vi "PRBS64 Parallel Tx Base.vi"(6 "ready for output (T)":bool=TRUE, 7 "reset":bool, 11 "seed":u64) -> (1 "output valid":bool, 3 "prbs tx":u64)   [LabVIEW 2022 SP3, in "Aurora64b66b Utilities FPGA.lvlib"]
uses:
  Aurora64b66b Utilities FPGA.lvlib
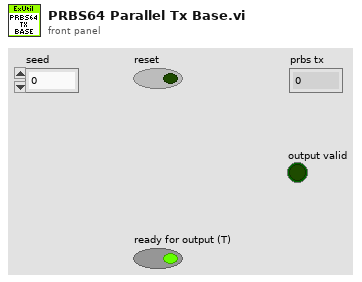
[diagram p1: front panel]
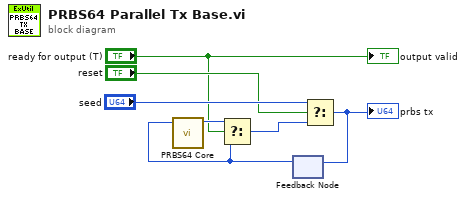
[diagram p0: block diagram]
diagram:
  n1 = feedback #1() -> (w4:u64)  [unwired: 1 in]
  n2 = call "PRBS64 Core.vi"("current value"=w4) -> ("next value"=w3:u64)  [unwired: 10 in]
  n3 = Select(t=w3, s="ready for output (T)", f=w4) -> (s? t:f=w2:u64)
  n4 = Select(t="seed", s="reset", f=w2) -> (s? t:f=w7:u64)
  "prbs tx" <- w7
  n5 = feedback-in #1(w7) -> ()
  "output valid" <- "ready for output (T)"
